vi "Initialize Settings.vi"(8 "error in (no error)":errorcluster, 10 "settings version":T3, 11 "settings":cluster{"key":string, "value":string}[](array[cluster])) -> (0 "error out":errorcluster, 3 "configuration":T1={"name"="Channel", "units"="V", "engine data type"=enum."DBL", "string data type"=enum."DBL", "string offset"=0} {"string offset" format="%d bytes"})   [LabVIEW 2017, in "DSF Core.lvlib" / "Core Channel Configuration.lvclass"]
uses:
  Core Channel Configuration.lvclass
  Typedefs/DSF Version Info.ctl
  Typedefs/DSF Core Channel Configuration.ctl
  Typedefs/DSF Data Type.ctl
  DSF Core.lvlib
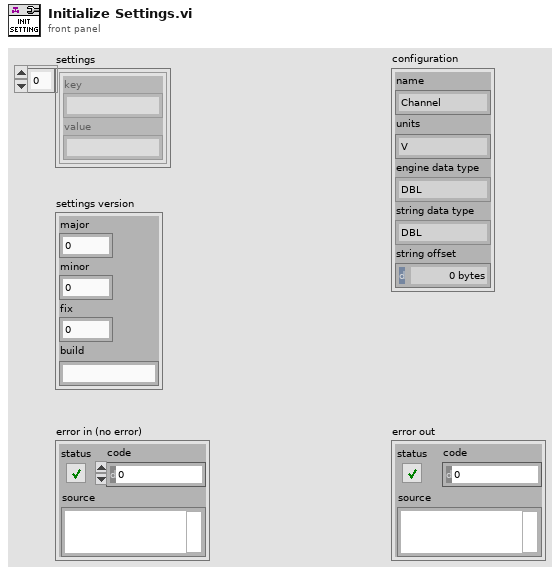
[diagram p1: front panel]
types:
  T1 = typedef "DSF Core.lvlib/DSF Core Channel Configuration.ctl" = cluster{"name":string, "units":string, "engine data type":T2, "string data type":T2, "string offset":u64}
  T2 = typedef "DSF Core.lvlib/DSF Data Type.ctl" = enum8{"Bool", "SGL", "DBL", "I8", "I16", "I32", "I64", "U8", "U16", "U32", "U64"}
  T3 = typedef "DSF Core.lvlib/DSF Version Info.ctl" = cluster{"major":u32, "minor":u32, "fix":u32, "build":string}
  T4 = cluster{"name":string, "units":string, "engine data type":enum8{"Bool", "SGL", "DBL", "I8", "I16", "I32", "I64", "U8", "U16", "U32", "U64"}, "string data type":enum8{"Bool", "SGL", "DBL", "I8", "I16", "I32", "I64", "U8", "U16", "U32", "U64"}, "string offset":u64}
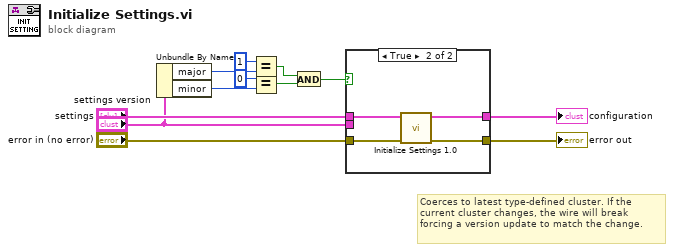
[diagram p0: block diagram]
diagram:
  # "Coerces to latest type-defined cluster. If the current cluster changes, the wire will break forcing a version update to match the change."
  n1 = Unbundle By Name("settings version") -> ("major"=w6:u32, "minor"=w9:u32)
  n2 = Equal?(x=u32 1, y=w6) -> (x = y?=w11:bool)
  n3 = Equal?(x=u32 0, y=w9) -> (x = y?=w10:bool)
  n4 = And(x=w11, y=w10) -> (x .and. y?=w12:bool)
  n5 = case shown="True" w12 {
    tunnel: "error in (no error)" -> [w13 w17]
    tunnel: [_ w14] -> w3
    tunnel: "settings" -> [_ w16]
    tunnel: [w13 w15] -> w5
    tunnel: "settings version" -> [_ _]
    frame False {
      # "Unknown version. Error."
    }
    frame True {
      n6 = call "Initialize Settings 1.0.vi"("error in (no error)"=w17, "settings 1.0"=w16) -> ("error out"=w15:errorcluster, "configuration 1.0"=w14:T4)  [unwired: 8 in]
    }
  }
  "error out" <- w5
  "configuration" <- w3
